vi "MovingAverage.vi"(10 "Rank":i32=15 min=1, 11 "Array in":dbl[](array[numeric])) -> (3 "Array out":dbl[](array[numeric]))   [LabVIEW 2013]
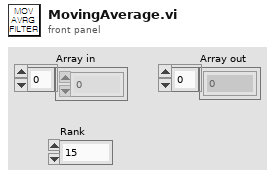
[diagram p1: front panel]
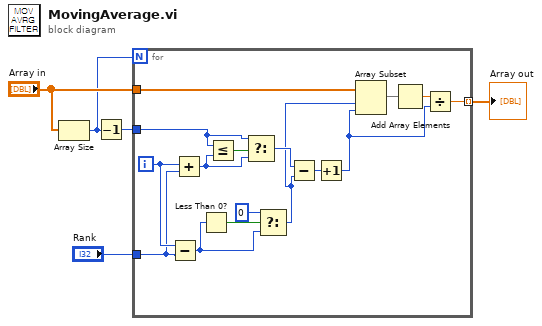
[diagram p0: block diagram]
diagram:
  n1 = Array Size(array="Array in") -> (size(s)=w2:i32)
  n2 = Decrement(x=w2) -> (x-1=w5:i32)
  n3 = for {
    N: w2 -> [_]
    tunnel: w5 -> [w15]
    tunnel: "Array in" -> [w11]
    tunnel: "Rank" -> [w17]
    tunnel: [w6] -> w1 mode=indexing
    i -> [w18]
    n4 = Subtract(x=w18, y=w17) -> (x-y=w19:i32)
    n5 = Add(x=w18, y=w17) -> (x+y=w14:i32)
    n6 = Less Than 0?(x=w19) -> (x < 0?=w20:bool)
    n7 = Less Or Equal?(x=w15, y=w14) -> (x <= y?=w16:bool)
    n8 = Select(t=w15, s=w16, f=w14) -> (s? t:f=w13:i32)
    n9 = Select(t=0, s=w20, f=w19) -> (s? t:f=w10:i32)
    n10 = Subtract(x=w13, y=w10) -> (x-y=w12:i32)
    n11 = Increment(x=w12) -> (x+1=w7:i32)
    n12 = Array Subset(array=w11, index=w10, length=w7) -> (w9:dbl[])
    n13 = Add Array Elements(numeric array=w9) -> (sum=w8:dbl)
    n14 = Divide(x=w8, y=w7) -> (x/y=w6:dbl)
  }
  "Array out" <- w1
